vi "SerialInit.vi"(3 "error in":errorcluster caption="错误输入", 4 "CAN通路":T1(ring), 5 "设备In":T2) -> (0 "error out":errorcluster caption="错误输出", 1 "VISAOut":refnum<visa-resource-name>, 2 "设备Out":T2)   [LabVIEW 2013]
uses:
  Ctl/DeviceCtl.ctl
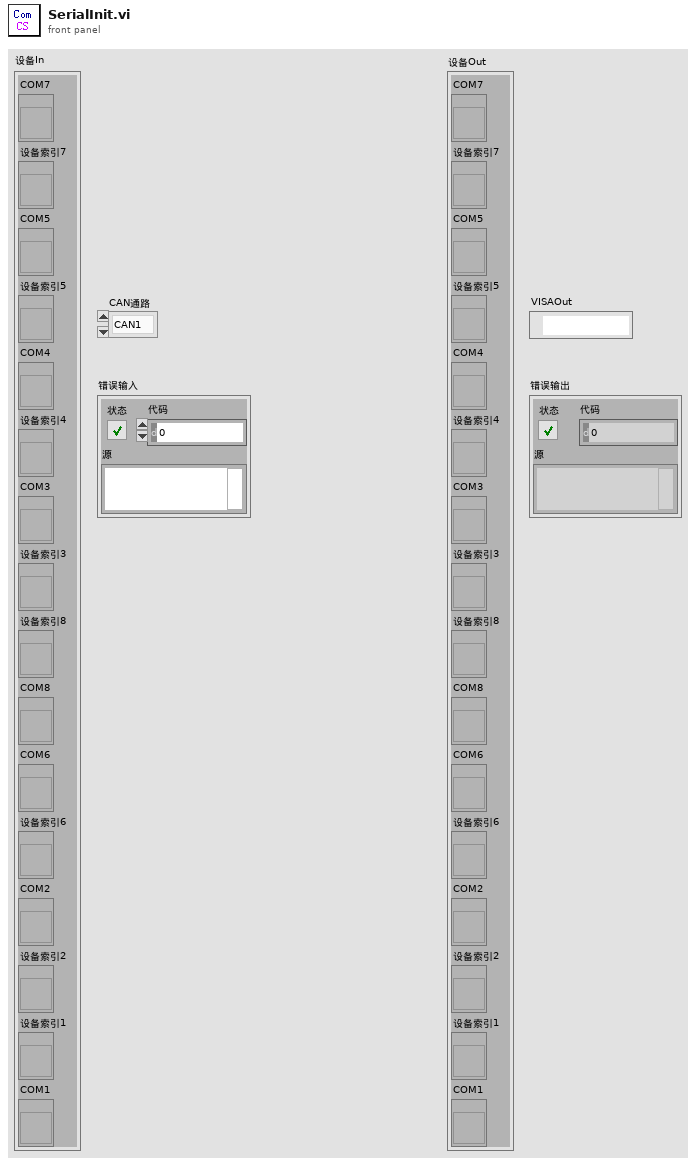
[diagram p1: front panel]
types:
  T1 = enum16{"CAN1", "CAN2", "CAN3", "CAN4", "CAN5", "CAN6", "CAN7", "CAN8"}
  T2 = typedef "DeviceCtl.ctl" = cluster{"COM7":refnum<vi>, "设备索引7":refnum<vi>, "COM5":refnum<vi>, "设备索引5":refnum<vi>, "COM4":refnum<vi>, "设备索引4":refnum<vi>, "COM3":refnum<vi>, "设备索引3":refnum<vi>, "设备索引8":refnum<vi>, "COM8":refnum<vi>, "COM6":refnum<vi>, "设备索引6":refnum<vi>, "COM2":refnum<vi>, "设备索引2":refnum<vi>, "设备索引1":refnum<vi>, "COM1":refnum<vi>}
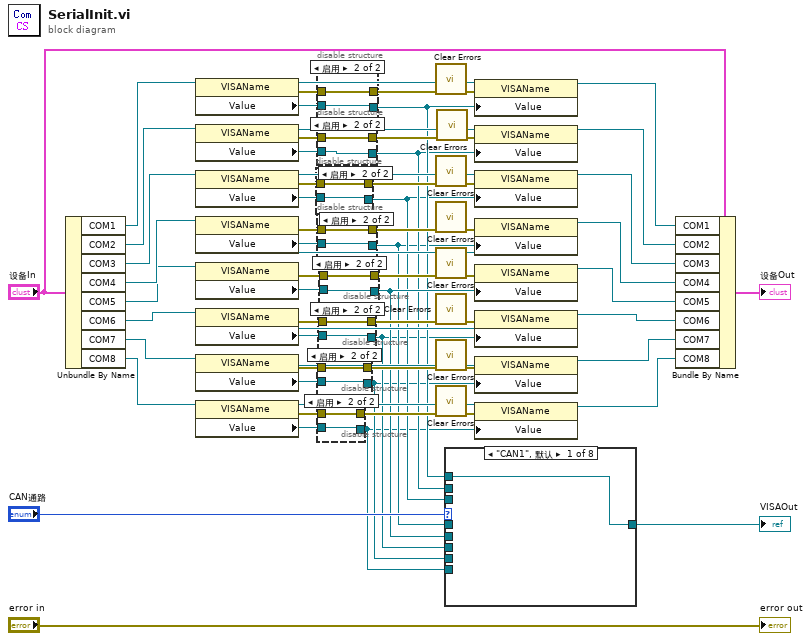
[diagram p0: block diagram]
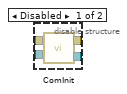
[diagram p2: hidden frame]
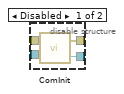
[diagram p3: hidden frame]
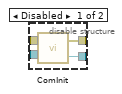
[diagram p4: hidden frame]
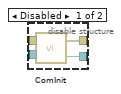
[diagram p5: hidden frame]
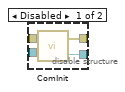
[diagram p6: hidden frame]
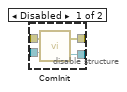
[diagram p7: hidden frame]
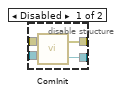
[diagram p8: hidden frame]
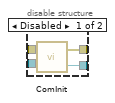
[diagram p9: hidden frame]
diagram:
  n1 = Unbundle By Name("设备In") -> ("COM1"=w69:refnum<vi>, "COM2"=w68:refnum<vi>, "COM3"=w67:refnum<vi>, "COM4"=w66:refnum<vi>, "COM5"=w65:refnum<vi>, "COM6"=w64:refnum<vi>, "COM7"=w63:refnum<vi>, "COM8"=w62:refnum<vi>)
  n2 = property class="VISAName"(reference=w69) -> (reference out=w36:refnum<vi>, error out=w61:errorcluster, "Value"=w60:refnum<visa-resource-name>)  [unwired: 1 in]
  n3 = property class="VISAName"(reference=w68) -> (reference out=w35:refnum<vi>, error out=w59:errorcluster, "Value"=w58:refnum<visa-resource-name>)  [unwired: 1 in]
  n4 = property class="VISAName"(reference=w67) -> (reference out=w34:refnum<vi>, error out=w57:errorcluster, "Value"=w56:refnum<visa-resource-name>)  [unwired: 1 in]
  n5 = property class="VISAName"(reference=w66) -> (reference out=w33:refnum<vi>, error out=w55:errorcluster, "Value"=w54:refnum<visa-resource-name>)  [unwired: 1 in]
  n6 = property class="VISAName"(reference=w65) -> (reference out=w32:refnum<vi>, error out=w53:errorcluster, "Value"=w52:refnum<visa-resource-name>)  [unwired: 1 in]
  n7 = property class="VISAName"(reference=w64) -> (reference out=w31:refnum<vi>, error out=w51:errorcluster, "Value"=w50:refnum<visa-resource-name>)  [unwired: 1 in]
  n8 = property class="VISAName"(reference=w63) -> (reference out=w30:refnum<vi>, error out=w49:errorcluster, "Value"=w48:refnum<visa-resource-name>)  [unwired: 1 in]
  n9 = property class="VISAName"(reference=w62) -> (reference out=w29:refnum<vi>, error out=w47:errorcluster, "Value"=w46:refnum<visa-resource-name>)  [unwired: 1 in]
  n10 = disable-structure shown="启用" {
    disable-tunnel: w57 -> [w73 w75]
    disable-tunnel: w56 -> [w72 w74]
    disable-tunnel: [w71 w75] -> w39
    disable-tunnel: [w70 w74] -> w15
    frame Disabled {
      n11 = call "ComInit.vi"("VISAIn"=w72, "error in"=w73) -> ("VISAOut"=w70:refnum<visa-resource-name>, "error out"=w71:errorcluster)
    }
    frame Enabled {
    }
  }
  n12 = disable-structure shown="启用" {
    disable-tunnel: w61 -> [w79 w81]
    disable-tunnel: w60 -> [w78 w80]
    disable-tunnel: [w77 w81] -> w37
    disable-tunnel: [w76 w80] -> w17
    frame Disabled {
      n13 = call "ComInit.vi"("VISAIn"=w78, "error in"=w79) -> ("VISAOut"=w76:refnum<visa-resource-name>, "error out"=w77:errorcluster)
    }
    frame Enabled {
    }
  }
  n14 = disable-structure shown="启用" {
    disable-tunnel: w59 -> [w85 w86]
    disable-tunnel: w58 -> [w84 w87]
    disable-tunnel: [w83 w86] -> w38
    disable-tunnel: [w82 w87] -> w16
    frame Disabled {
      n15 = call "ComInit.vi"("VISAIn"=w84, "error in"=w85) -> ("VISAOut"=w82:refnum<visa-resource-name>, "error out"=w83:errorcluster)
    }
    frame Enabled {
    }
  }
  n16 = disable-structure shown="启用" {
    disable-tunnel: w55 -> [w91 w93]
    disable-tunnel: w54 -> [w90 w92]
    disable-tunnel: [w89 w93] -> w40
    disable-tunnel: [w88 w92] -> w14
    frame Disabled {
      n17 = call "ComInit.vi"("VISAIn"=w90, "error in"=w91) -> ("VISAOut"=w88:refnum<visa-resource-name>, "error out"=w89:errorcluster)
    }
    frame Enabled {
    }
  }
  n18 = disable-structure shown="启用" {
    disable-tunnel: w49 -> [w97 w99]
    disable-tunnel: w48 -> [w96 w98]
    disable-tunnel: [w95 w99] -> w43
    disable-tunnel: [w94 w98] -> w11
    frame Disabled {
      n19 = call "ComInit.vi"("VISAIn"=w96, "error in"=w97) -> ("VISAOut"=w94:refnum<visa-resource-name>, "error out"=w95:errorcluster)
    }
    frame Enabled {
    }
  }
  n20 = disable-structure shown="启用" {
    disable-tunnel: w47 -> [w103 w105]
    disable-tunnel: w46 -> [w102 w104]
    disable-tunnel: [w101 w105] -> w44
    disable-tunnel: [w100 w104] -> w10
    frame Disabled {
      n21 = call "ComInit.vi"("VISAIn"=w102, "error in"=w103) -> ("VISAOut"=w100:refnum<visa-resource-name>, "error out"=w101:errorcluster)
    }
    frame Enabled {
    }
  }
  n22 = disable-structure shown="启用" {
    disable-tunnel: w51 -> [w109 w111]
    disable-tunnel: w50 -> [w108 w110]
    disable-tunnel: [w107 w111] -> w42
    disable-tunnel: [w106 w110] -> w12
    frame Disabled {
      n23 = call "ComInit.vi"("VISAIn"=w108, "error in"=w109) -> ("VISAOut"=w106:refnum<visa-resource-name>, "error out"=w107:errorcluster)
    }
    frame Enabled {
    }
  }
  n24 = disable-structure shown="启用" {
    disable-tunnel: w53 -> [w115 w117]
    disable-tunnel: w52 -> [w114 w116]
    disable-tunnel: [w113 w117] -> w41
    disable-tunnel: [w112 w116] -> w13
    frame Disabled {
      n25 = call "ComInit.vi"("VISAIn"=w114, "error in"=w115) -> ("VISAOut"=w112:refnum<visa-resource-name>, "error out"=w113:errorcluster)
    }
    frame Enabled {
    }
  }
  n26 = call <vilib>:"Clear Errors.vi"("error in (no error)"=w37) -> ("error out"=w8:errorcluster)  [unwired: 6 in]
  n27 = call <vilib>:"Clear Errors.vi"("error in (no error)"=w39) -> ("error out"=w6:errorcluster)  [unwired: 6 in]
  n28 = call <vilib>:"Clear Errors.vi"("error in (no error)"=w40) -> ("error out"=w5:errorcluster)  [unwired: 6 in]
  n29 = call <vilib>:"Clear Errors.vi"("error in (no error)"=w41) -> ("error out"=w4:errorcluster)  [unwired: 6 in]
  n30 = call <vilib>:"Clear Errors.vi"("error in (no error)"=w42) -> ("error out"=w3:errorcluster)  [unwired: 6 in]
  n31 = call <vilib>:"Clear Errors.vi"("error in (no error)"=w43) -> ("error out"=w2:errorcluster)  [unwired: 6 in]
  n32 = call <vilib>:"Clear Errors.vi"("error in (no error)"=w44) -> ("error out"=w1:errorcluster)  [unwired: 6 in]
  n33 = call <vilib>:"Clear Errors.vi"("error in (no error)"=w38) -> ("error out"=w7:errorcluster)  [unwired: 6 in]
  n34 = case shown="\"CAN1\", 默认" "CAN通路" {
    tunnel: w17 -> [w118 _ _ _ _ _ _ _]
    tunnel: w16 -> [_ w119 _ _ _ _ _ _]
    tunnel: w15 -> [_ _ w120 _ _ _ _ _]
    tunnel: w14 -> [_ _ _ w121 _ _ _ _]
    tunnel: w13 -> [_ _ _ _ w122 _ _ _]
    tunnel: w12 -> [_ _ _ _ _ w123 _ _]
    tunnel: w11 -> [_ _ _ _ _ _ w124 _]
    tunnel: w10 -> [_ _ _ _ _ _ _ w125]
    tunnel: [w118 w119 w120 w121 w122 w123 w124 w125] -> w9
    frame "CAN1", Default {
    }
    frame "CAN2" {
    }
    frame "CAN3" {
    }
    frame "CAN4" {
    }
    frame "CAN5" {
    }
    frame "CAN6" {
    }
    frame "CAN7" {
    }
    frame "CAN8" {
    }
  }
  "VISAOut" <- w9
  n35 = property class="VISAName"(reference=w36, error in=w8, "Value"=w17) -> (reference out=w28:refnum<vi>)  [unwired: 1 out]
  n36 = property class="VISAName"(reference=w35, error in=w7, "Value"=w16) -> (reference out=w27:refnum<vi>)  [unwired: 1 out]
  n37 = property class="VISAName"(reference=w34, error in=w6, "Value"=w15) -> (reference out=w26:refnum<vi>)  [unwired: 1 out]
  n38 = property class="VISAName"(reference=w33, error in=w5, "Value"=w14) -> (reference out=w25:refnum<vi>)  [unwired: 1 out]
  n39 = property class="VISAName"(reference=w32, error in=w4, "Value"=w13) -> (reference out=w24:refnum<vi>)  [unwired: 1 out]
  n40 = property class="VISAName"(reference=w31, error in=w3, "Value"=w12) -> (reference out=w23:refnum<vi>)  [unwired: 1 out]
  n41 = property class="VISAName"(reference=w30, error in=w2, "Value"=w11) -> (reference out=w22:refnum<vi>)  [unwired: 1 out]
  n42 = property class="VISAName"(reference=w29, error in=w1, "Value"=w10) -> (reference out=w21:refnum<vi>)  [unwired: 1 out]
  n43 = Bundle By Name(cluster="设备In", "COM1"=w28, "COM2"=w27, "COM3"=w26, "COM4"=w25, "COM5"=w24, "COM6"=w23, "COM7"=w22, "COM8"=w21) -> (→"设备Out":T2)
  "error out" <- "error in"
